vi "digital_demod_host.vi"() -> ()   [LabVIEW 2014]
uses:
  <vilib>/userdefined/High Color/nirio_resource_hc.ctl
  <vilib>/LabVIEW Targets/FPGA/RIO/nirio_PxiTriggers.ctl
  <vilib>/addons/h5labview2/file/H5Fmode.ctl
  <vilib>/FPGAPlugInAG/PXI-7854R/niLvFpga_Open_PXI-7854R.vi
  <vilib>/rvi/interface/common/dynamic/niFpgaDynamicAddResources.vi
  <vilib>/FPGAPlugInAG/Dynamic/niLvFpga_Run_Dynamic.vi
  <vilib>/LabVIEW Targets/FPGA/RIO/nirioReserveTrigger.vi
  <vilib>/Utility/error.llb/Error Cluster From Error Code.vi
  <vilib>/rvi/errors/niLvFpgaAdjustHostInterfaceError.vi
  <vilib>/addons/h5labview2/base/lib_path.vi
  <vilib>/addons/h5labview2/base/H5Equery.vi
  <vilib>/FPGAPlugInAG/Dynamic/niLvFpga_Close_Dynamic.vi
  <vilib>/rvi/interface/nirviOpenFPGA/nirviOpenFPGA.xnode
  FPGA Bitfiles/digitaldemod_FPGATarget_digitaldemodfpga_GJzl1kj7Fe4.lvbitx
  <vilib>/rvi/interface/nirviMethod/nirviMethod.xnode
  <vilib>/rvi/interface/nirviReadWriteControl/nirviReadWriteControl.xnode
  <vilib>/addons/h5labview2/base/hid_t.ctl
  <vilib>/addons/h5labview2/dataset/H5Dwrite.llb/H5Dwrite.xnode
  <vilib>/rvi/interface/nirviCloseFPGA/nirviCloseFPGA.xnode
  <vilib>/rvi/interface/Simulation/niFpgaSimulationCallBeginRW.vi
  <vilib>/rvi/errors/niLvFpgaMergeErrorWithErrorCode.vi
  <vilib>/FPGAPlugInAG/Dynamic/niLvFpga_ReadFifo_Dynamic.vi
  NiFpgaLv.dll
  <vilib>/addons/h5labview2/group/H5G.lvlib
  <vilib>/addons/h5labview2/file/H5F.lvlib
  <vilib>/FPGAPlugInAG/Dynamic/niLvFpga_StartFifo_Dynamic.vi
  <vilib>/FPGAPlugInAG/Dynamic/niLvFpga_StopFifo_Dynamic.vi
  National Instruments Downloads/LabVIEW FPGA English/FPGA Timekeeper 1.1b0/FPGA Timekeeper.lvlib
panel:
  in  "show_quad":bool
  out "delta_phi":cluster{dbl, dbl, dbl, dbl}(graph)
  in  "xy2_bitshift":i16
  in  "downsample->xyz":bool
  in  "inject_sigs":bool
  in  "Load last pars":bool
  in  "DAQ_trig":bool
  in  "Reset Phi 2":bool
  in  "reset_z_accum":bool
  out "config_trig":bool
  in  "block_hardware_trigs":bool=TRUE
  out "config_loaded":bool
  out "Nsamp_config":u32=50000
  out "fpga_dat_path":path=path "C:/Data/20180611/bead6/post_pump/turbombar_xyzcool_pumped_0_fpga.h5"
  in  "reset_trigs":bool
  in  "accept_trigs":bool
  out "amp4":dbl(graph)=1893.4088287353516
  out "phi4":dbl(graph)=0.028564453125
  in  "Change Pars 2":bool
  in  "xy_fb_bitshift":i16=-13
  in  "z_lower_lim":i16=-2000
  in  "z_upper_lim":i16=2000
  in  "z_fb_bitshift":i16=-16
  in  "z_ig":fxp<+/-,32,16>=-1.52587890625e-05
  in  "z_dg":fxp<+/-,32,16>=-0.0500640869140625
  in  "z_pg":fxp<+/-,32,16>=-0.0099945068359375
  in  "z_bitshift":i16
  in  "y_lower_lim":i16=-1000
  in  "y_upper_lim":i16=1000
  in  "y_dg":fxp<+/-,32,16>=-0.0019989013671875
  in  "x_lower_lim":i16=-1000
  in  "x_upper_lim":i16=1000
  in  "x_dg":fxp<+/-,32,16>=0.001007080078125
  in  "xy_bitshift":i16=-13
  in  "read_raw":bool
  out "z_fb":i16(graph)=-749
  out "z":i32(graph)=551
  out "y_fb":i16(graph)=2
  out "y":i32(graph)=-854
  out "x_fb":i16(graph)=-1
  out "x":i32(graph)=4640
  in  "z_set":fxp<+/-,32,32>
  in  "z_dc_offset":i16=-17500
  in  "y_dc_offset":i16
  in  "x_dc_offset":i16
  out "Host time (ns)":u64=1528843412913566976
  out "Target time (ns)":u64=1528843412913588017
  in  "downsamp_num":i16=100
  in  "Reset Phi Params":T1={"All Phi?"=TRUE, "Which?"=enum."0"}
  out "amp2":dbl(graph)=9755.388763427734
  out "amp3":dbl(graph)=9270.060470581055
  out "amp0":dbl(graph)=9360.88851928711
  out "amp1":dbl(graph)=10535.541046142578
  out "phi2":dbl(graph)=-7.1851806640625
  out "phi3":dbl(graph)=-7.253662109375
  in  "subtract_mean":bool=TRUE
  out "loop time":fxp<+,32,32>=2.0
  in  "Change Pars":bool
  out "phi0":dbl(graph)=-6.774658203125
  out "phi1":dbl(graph)=-6.8974609375
  in  "counter offset":u32
  in  "phase discont_neg":fxp<+/-,24,12>=-1.0
  in  "phase discont_pos":fxp<+/-,24,12>=1.0
  in  "Reset Phi":bool
  in  "loop timer (usec)":u32=2
  in  "Update ADC Clock":bool
  in  "Host Update Rate (msec)":dbl=1.0 format="%#_13g"
  in  "RIO Device":T2="RIO0"
  # "QPD AMPLITUDES"
  # "QPD PHASES"
  # "BACKSCATTER"
  # "BEAD XYZ + FB"
  # "X FEEDBACK"
  # "Y FEEDBACK"
  # "Z FEEDBACK"
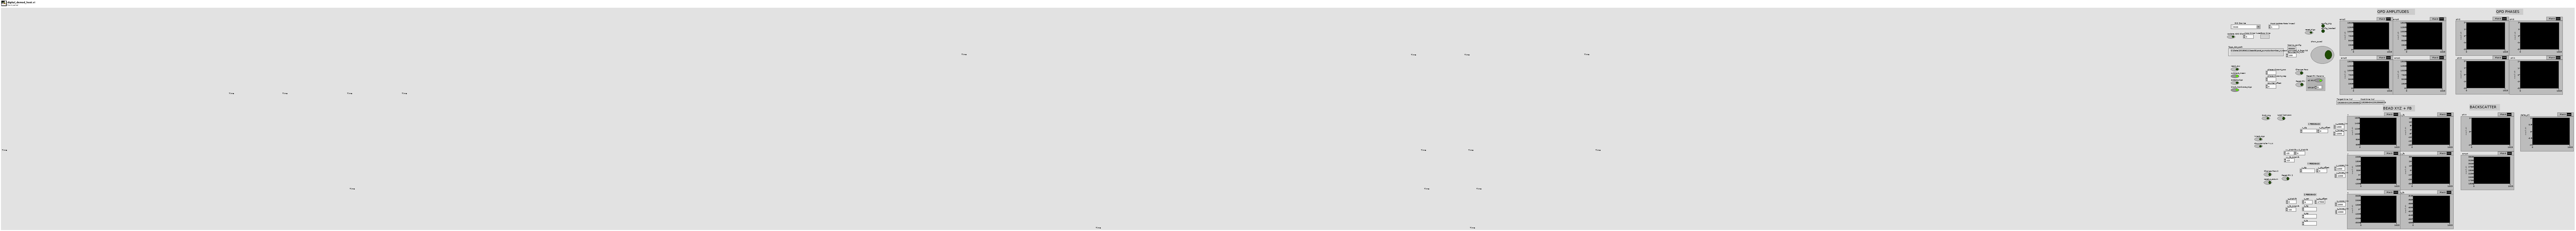
[diagram p1: front panel]
types:
  T1 = cluster{"All Phi?":bool, "Which?":enum16{"0", "1", "2", "3", "4"}}
  T2 = typedef "nirio_resource_hc.ctl" = tag
  T3 = typedef "nirio_PxiTriggers.ctl" = u16
  T4 = cluster{"phase discont_pos":fxp<+/-,24,12>, "phase discont_neg":fxp<+/-,24,12>, "counter offset":u32, "subtract_mean":bool, "downsamp_num":i16, "xy_bitshift":i16, "x_dg":fxp<+/-,32,16>, "x_upper_lim":i16, "x_lower_lim":i16, "x_dc_offset":i16, "y_dg":fxp<+/-,32,16>, "y_upper_lim":i16, "y_lower_lim":i16, "y_dc_offset":i16, "xy_fb_bitshift":i16, "z_bitshift":i16, "z_set":fxp<+/-,32,32>, "z_pg":fxp<+/-,32,16>, "z_dg":fxp<+/-,32,16>, "z_ig":fxp<+/-,32,16>, "z_fb_bitshift":i16, "z_upper_lim":i16, "z_lower_lim":i16, "z_dc_offset":i16, "inject_sigs":bool, "downsample->xyz":bool, "xy2_bitshift":i16}
  T5 = enum16{"open", "replace", "create", "open or create", "replace or create", "replace or create with confirmation"}
  T6 = typedef "H5F.lvlib/H5Fmode.ctl" = enum16{"read-only", "read-write", "overwrite", "create new", "open or create"}
  T7 = typedef "hid_t.ctl" = i32
  T8 = cluster{fxp<+/-,33,19>, fxp<+/-,33,19>, fxp<+/-,33,19>, fxp<+/-,33,19>}
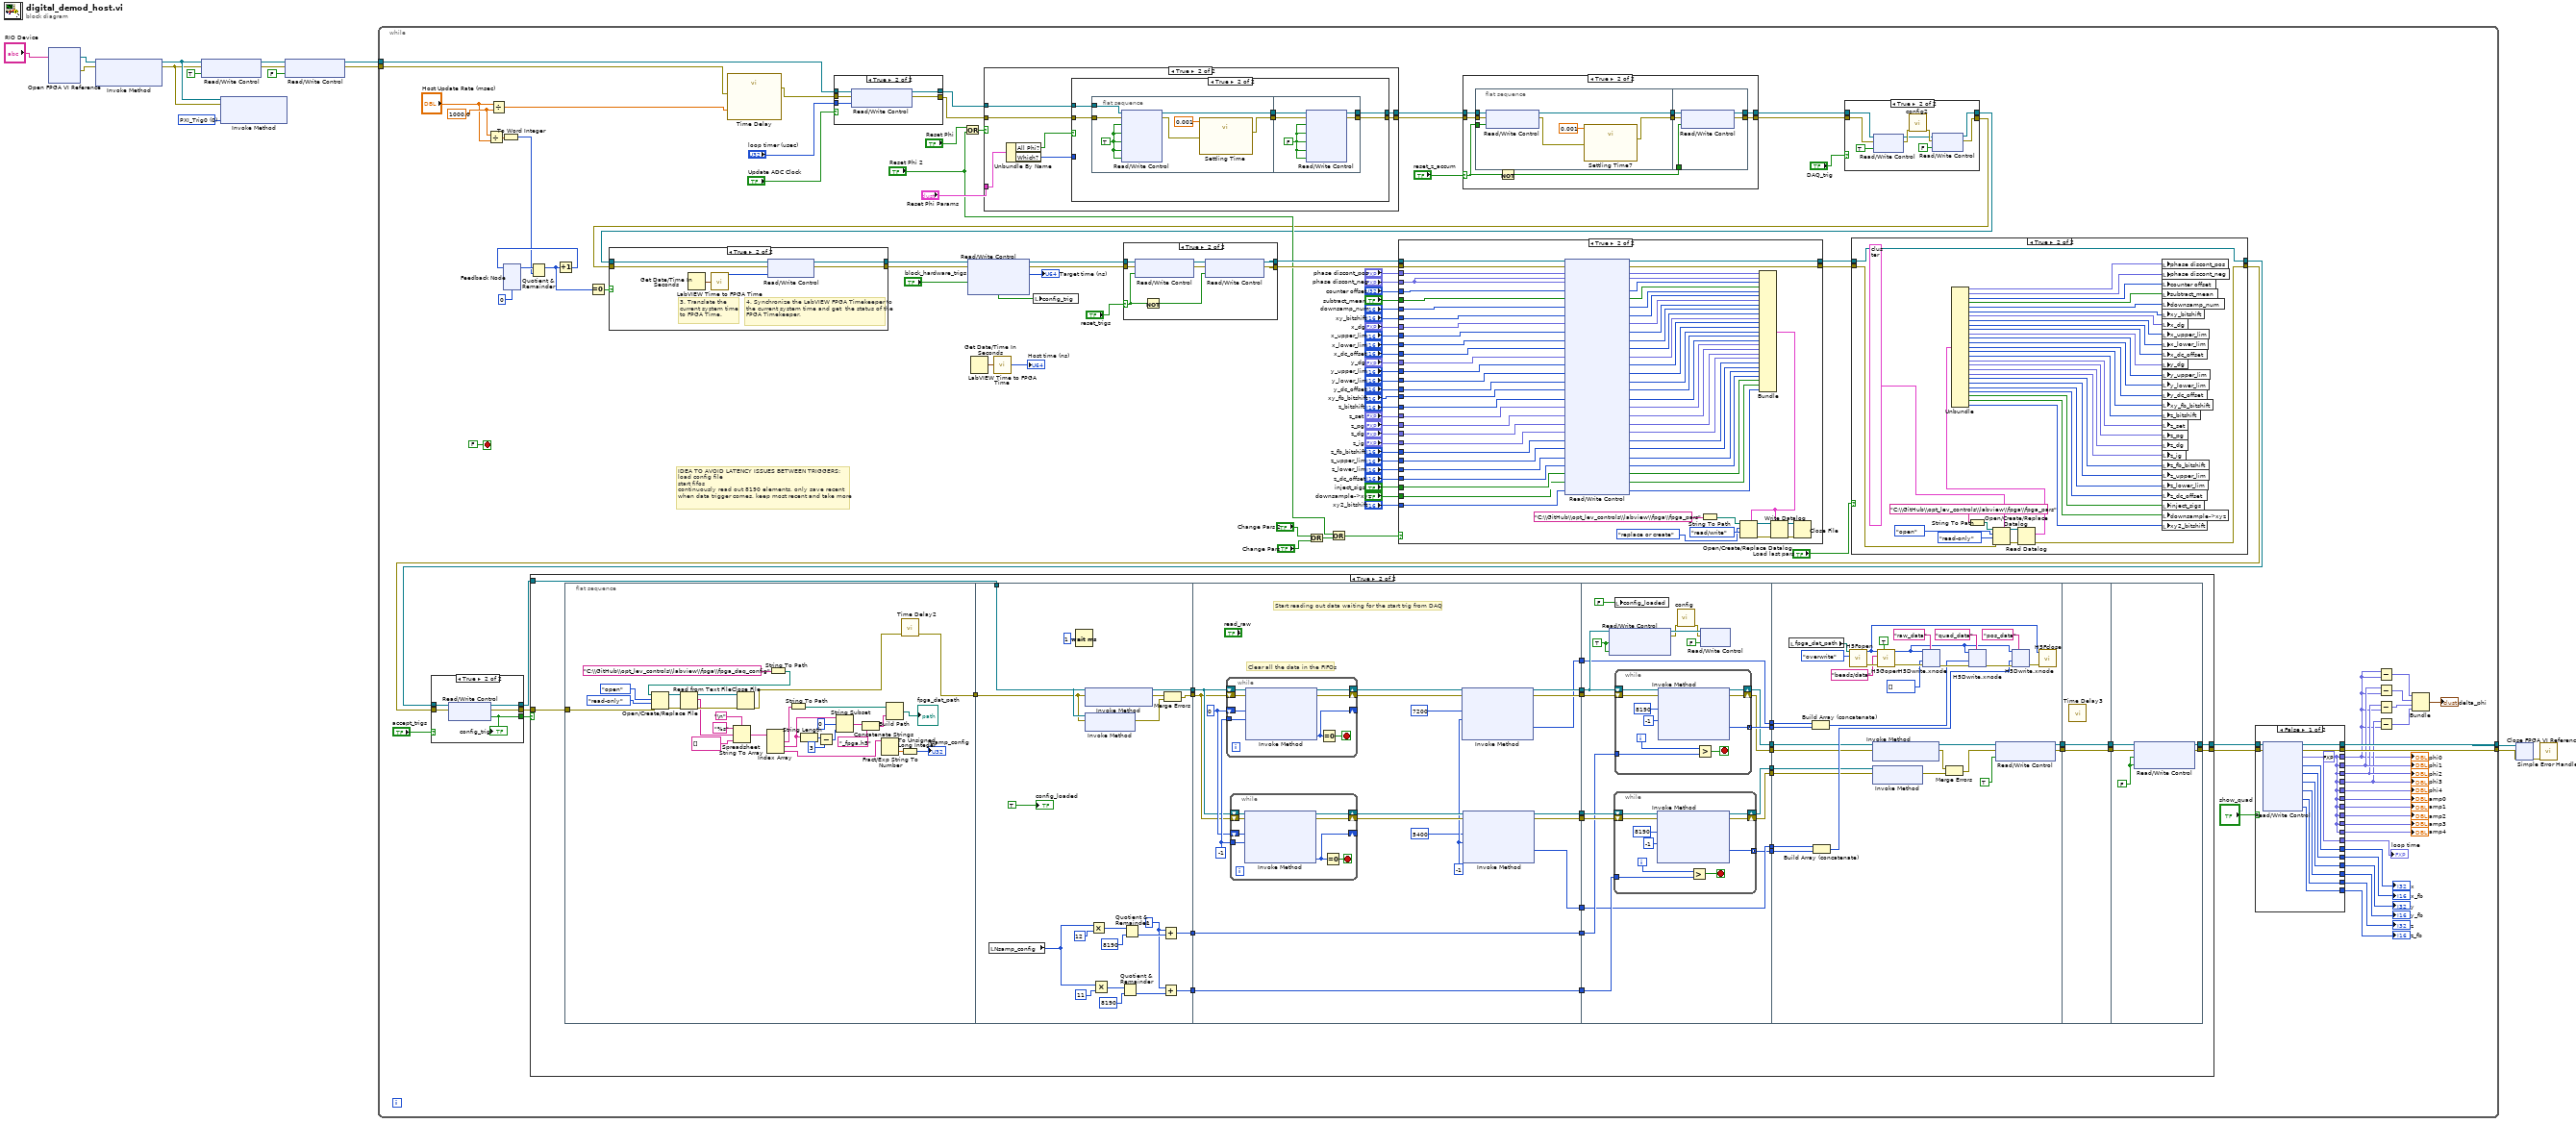
[diagram p0: block diagram]
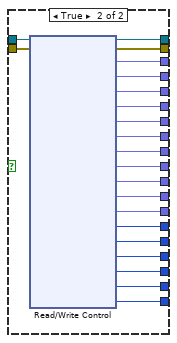
[diagram p2: hidden frame]
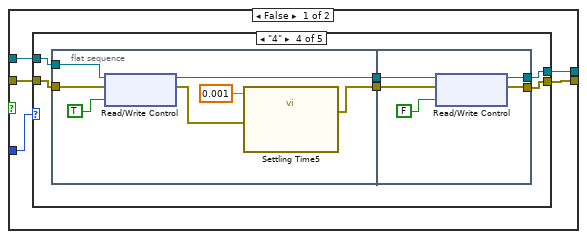
[diagram p12: hidden frame]
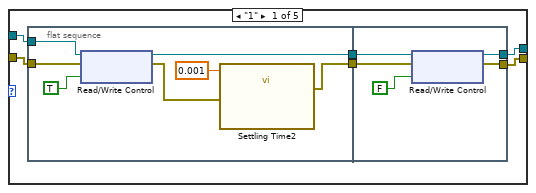
[diagram p13: hidden frame]
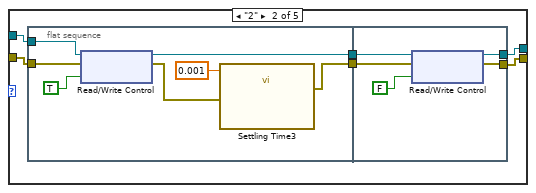
[diagram p14: hidden frame]
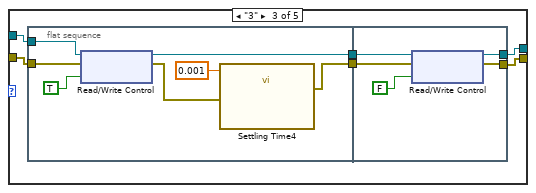
[diagram p15: hidden frame]
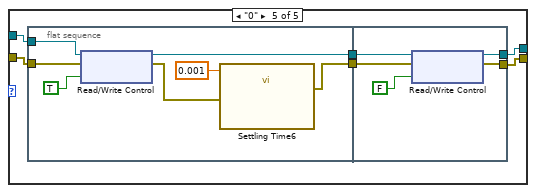
[diagram p16: hidden frame]
diagram:
  w1 = T3 0 items=["PXI_Trig0", "PXI_Trig1", "PXI_Trig2", "PXI_Trig3", "PXI_Trig4", "PXI_Trig5", "PXI_Trig6", "PXI_Trig7"] ("Trigger")
  n1 = xnode "Open FPGA VI Reference"("resource name"="RIO Device") -> ("FPGA VI Reference Out"=w11:refnum<k20>, "error out"=w10:errorcluster)  [unwired: 1 in]
  n2 = xnode "Invoke Method"("FPGA VI Reference In"=w11, "error in"=w10) -> ("FPGA VI Reference Out"=w3:refnum<k20>, "error out"=w2:errorcluster)  [unwired: 1 in]
  n3 = xnode "Read/Write Control"("FPGA VI Reference In"=w3, "error in"=w2, "reset_config_trig"=TRUE ("reset_trig")) -> ("FPGA VI Reference Out"=w6:refnum<k20>, "error out"=w4:errorcluster)
  n4 = xnode "Invoke Method"("FPGA VI Reference In"=w3, "error in"=w2, "Trigger"=w1) -> ()  [unwired: 2 out]
  n5 = xnode "Read/Write Control"("FPGA VI Reference In"=w6, "error in"=w4, "reset_config_trig"=FALSE ("manual_trig")) -> ("FPGA VI Reference Out"=w9:refnum<k20>, "error out"=w8:errorcluster)
  n6 = while {
    tunnel: w8 -> [w123]
    tunnel: w9 -> [w39]
    tunnel: [w114] -> w14
    tunnel: [w113] -> w13
    stop <- FALSE stop-if-true
    w104 = 1000.0
    # "IDEA TO AVOID LATENCY ISSUES BETWEEN TRIGGERS:\nload config file\nstart fifos\ncontinuously read out 8190 elements, only save recent\nwhen data trigger comes, keep most recent and take more"
    n7 = Divide(x=w104, y="Host Update Rate (msec)") -> (x/y=w102:dbl)
    n8 = Divide(x="Host Update Rate (msec)", y=w104) -> (x/y=w124:dbl)
    n9 = To Word Integer(number=w102) -> (16bit integer=w96:i16)
    n10 = feedback #1(i16 0) -> (w98:i16)
    n11 = Quotient & Remainder(x=w98, y=w96) -> (x-y*floor(x/y)=w95:i16)  [unwired: 1 out]
    n12 = Increment(x=w95) -> (x+1=w97:i16)
    n13 = feedback-in #1(w97) -> ()
    n14 = Equal To 0?(x=w95) -> (x = 0?=w100:bool)
    n15 = call "Time Delay"("error in (no error)"=w123, "Delay Time (s)"=w124) -> ("error out"=w121:errorcluster)  [unwired: 9 in]
    n16 = case shown="True" "Update ADC Clock" {
      tunnel: w39 -> [w671 w676]
      tunnel: w121 -> [w670 w675]
      tunnel: [w671 w674] -> w119
      tunnel: [w670 w673] -> w118
      tunnel: "loop timer (usec)" -> [_ w672]
      frame False {
      }
      frame True {
        n17 = xnode "Read/Write Control"("FPGA VI Reference In"=w676, "error in"=w675, "loop timer (usec)"=w672) -> ("FPGA VI Reference Out"=w674:refnum<k20>, "error out"=w673:errorcluster)
      }
    }
    n18 = Or(x="Reset Phi", y="Reset Phi 2") -> (x .or. y?=w45:bool)
    n19 = Get Date/Time In Seconds() -> (seconds since 1Jan1904=w93:timestamp)
    n20 = case shown="True" w45 {
      tunnel: w119 -> [w549 w556]
      tunnel: w118 -> [w548 w555]
      tunnel: [w549 w553] -> w48
      tunnel: [w548 w554] -> w47
      tunnel: "Reset Phi Params" -> [_ w552]
      frame False {
      }
      frame True {
        n21 = Unbundle By Name(w552) -> ("All Phi?"=w551:bool, "Which?"=w550:enum16{"0", "1", "2", "3", "4"})
        n22 = case shown="True" w551 {
          tunnel: w556 -> [w561 w655]
          tunnel: w555 -> [w560 w654]
          tunnel: [w558 w653] -> w554
          tunnel: [w559 w652] -> w553
          tunnel: w550 -> [w557 _]
          frame False {
            n23 = case shown="\"4\"" w557 {
              tunnel: w561 -> [w565 w583 w601 w619 w637]
              tunnel: w560 -> [w564 w582 w600 w618 w636]
              tunnel: [w563 w581 w599 w617 w635] -> w559
              tunnel: [w562 w580 w598 w616 w634] -> w558
              frame "1" {
                n24 = flat-sequence {
                  tunnel: w565 -> [w574]
                  tunnel: w564 -> [w573]
                  tunnel: [w572] -> w567
                  tunnel: [w569] -> w566
                  tunnel: w567 -> [w579]
                  tunnel: w566 -> [w578]
                  tunnel: [w577] -> w563
                  tunnel: [w576] -> w562
                  frame #0 {
                    n25 = xnode "Read/Write Control"("FPGA VI Reference In"=w574, "error in"=w573, "reset_phi1"=TRUE) -> ("FPGA VI Reference Out"=w572:refnum<k20>, "error out"=w570:errorcluster)
                    n26 = call "Settling Time2"("error in (no error)"=w570, "Delay Time (s)"=0.001) -> ("error out"=w569:errorcluster)  [unwired: 9 in]
                  }
                  frame #1 {
                    n27 = xnode "Read/Write Control"("FPGA VI Reference In"=w579, "error in"=w578, "reset_phi1"=FALSE) -> ("FPGA VI Reference Out"=w577:refnum<k20>, "error out"=w576:errorcluster)
                  }
                }
              }
              frame "2" {
                n28 = flat-sequence {
                  tunnel: w583 -> [w592]
                  tunnel: w582 -> [w591]
                  tunnel: [w590] -> w585
                  tunnel: [w587] -> w584
                  tunnel: w585 -> [w597]
                  tunnel: w584 -> [w596]
                  tunnel: [w595] -> w581
                  tunnel: [w594] -> w580
                  frame #0 {
                    n29 = xnode "Read/Write Control"("FPGA VI Reference In"=w592, "error in"=w591, "reset_phi2"=TRUE) -> ("FPGA VI Reference Out"=w590:refnum<k20>, "error out"=w588:errorcluster)
                    n30 = call "Settling Time3"("error in (no error)"=w588, "Delay Time (s)"=0.001) -> ("error out"=w587:errorcluster)  [unwired: 9 in]
                  }
                  frame #1 {
                    n31 = xnode "Read/Write Control"("FPGA VI Reference In"=w597, "error in"=w596, "reset_phi2"=FALSE) -> ("FPGA VI Reference Out"=w595:refnum<k20>, "error out"=w594:errorcluster)
                  }
                }
              }
              frame "3" {
                n32 = flat-sequence {
                  tunnel: w601 -> [w610]
                  tunnel: w600 -> [w609]
                  tunnel: [w608] -> w603
                  tunnel: [w605] -> w602
                  tunnel: w603 -> [w615]
                  tunnel: w602 -> [w614]
                  tunnel: [w613] -> w599
                  tunnel: [w612] -> w598
                  frame #0 {
                    n33 = xnode "Read/Write Control"("FPGA VI Reference In"=w610, "error in"=w609, "reset_phi3"=TRUE) -> ("FPGA VI Reference Out"=w608:refnum<k20>, "error out"=w606:errorcluster)
                    n34 = call "Settling Time4"("error in (no error)"=w606, "Delay Time (s)"=0.001) -> ("error out"=w605:errorcluster)  [unwired: 9 in]
                  }
                  frame #1 {
                    n35 = xnode "Read/Write Control"("FPGA VI Reference In"=w615, "error in"=w614, "reset_phi3"=FALSE) -> ("FPGA VI Reference Out"=w613:refnum<k20>, "error out"=w612:errorcluster)
                  }
                }
              }
              frame "4" {
                n36 = flat-sequence {
                  tunnel: w619 -> [w628]
                  tunnel: w618 -> [w627]
                  tunnel: [w626] -> w621
                  tunnel: [w623] -> w620
                  tunnel: w621 -> [w633]
                  tunnel: w620 -> [w632]
                  tunnel: [w631] -> w617
                  tunnel: [w630] -> w616
                  frame #0 {
                    n37 = xnode "Read/Write Control"("FPGA VI Reference In"=w628, "error in"=w627, "reset_phi4"=TRUE) -> ("FPGA VI Reference Out"=w626:refnum<k20>, "error out"=w624:errorcluster)
                    n38 = call "Settling Time5"("error in (no error)"=w624, "Delay Time (s)"=0.001) -> ("error out"=w623:errorcluster)  [unwired: 9 in]
                  }
                  frame #1 {
                    n39 = xnode "Read/Write Control"("FPGA VI Reference In"=w633, "error in"=w632, "reset_phi4"=FALSE) -> ("FPGA VI Reference Out"=w631:refnum<k20>, "error out"=w630:errorcluster)
                  }
                }
              }
              frame "0" {
                n40 = flat-sequence {
                  tunnel: w637 -> [w646]
                  tunnel: w636 -> [w645]
                  tunnel: [w644] -> w639
                  tunnel: [w641] -> w638
                  tunnel: w639 -> [w651]
                  tunnel: w638 -> [w650]
                  tunnel: [w649] -> w635
                  tunnel: [w648] -> w634
                  frame #0 {
                    n41 = xnode "Read/Write Control"("FPGA VI Reference In"=w646, "error in"=w645, "reset_phi0"=TRUE) -> ("FPGA VI Reference Out"=w644:refnum<k20>, "error out"=w642:errorcluster)
                    n42 = call "Settling Time6"("error in (no error)"=w642, "Delay Time (s)"=0.001) -> ("error out"=w641:errorcluster)  [unwired: 9 in]
                  }
                  frame #1 {
                    n43 = xnode "Read/Write Control"("FPGA VI Reference In"=w651, "error in"=w650, "reset_phi0"=FALSE) -> ("FPGA VI Reference Out"=w649:refnum<k20>, "error out"=w648:errorcluster)
                  }
                }
              }
            }
          }
          frame True {
            n44 = flat-sequence {
              tunnel: w655 -> [w664]
              tunnel: w654 -> [w663]
              tunnel: [w662] -> w657
              tunnel: [w659] -> w656
              tunnel: w657 -> [w669]
              tunnel: w656 -> [w668]
              tunnel: [w667] -> w652
              tunnel: [w666] -> w653
              frame #0 {
                w658 = TRUE
                n45 = xnode "Read/Write Control"("FPGA VI Reference In"=w664, "error in"=w663, "reset_phi0"=w658, "reset_phi1"=w658, "reset_phi2"=w658, "reset_phi3"=w658, "reset_phi4"=w658) -> ("FPGA VI Reference Out"=w662:refnum<k20>, "error out"=w660:errorcluster)
                n46 = call "Settling Time"("error in (no error)"=w660, "Delay Time (s)"=0.001) -> ("error out"=w659:errorcluster)  [unwired: 9 in]
              }
              frame #1 {
                w665 = FALSE
                n47 = xnode "Read/Write Control"("FPGA VI Reference In"=w669, "error in"=w668, "reset_phi0"=w665, "reset_phi1"=w665, "reset_phi2"=w665, "reset_phi3"=w665, "reset_phi4"=w665) -> ("FPGA VI Reference Out"=w667:refnum<k20>, "error out"=w666:errorcluster)
              }
            }
          }
        }
      }
    }
    n48 = call "LabVIEW Time to FPGA Time.vi"("LabVIEW time"=w93) -> ("FPGA time (ns)"=→"Host time (ns)":u64)
    n49 = Or(x="Change Pars 2", y="Change Pars") -> (x .or. y?=w43:bool)
    n50 = Or(x="Reset Phi 2", y=w43) -> (x .or. y?=w42:bool)
    n51 = case shown="True" "reset_z_accum" {
      selector: "reset_z_accum" -> [_ w212]
      tunnel: w48 -> [w210 w218]
      tunnel: w47 -> [w209 w217]
      tunnel: [w210 w216] -> w37
      tunnel: [w209 w215] -> w36
      frame False {
      }
      frame True {
        n52 = flat-sequence {
          tunnel: w218 -> [w225]
          tunnel: w217 -> [w224]
          tunnel: w212 -> [w222]
          tunnel: [w223] -> w214
          tunnel: [w219] -> w213
          tunnel: [w227] -> w215
          tunnel: [w228] -> w216
          tunnel: w214 -> [w230]
          tunnel: w213 -> [w229]
          tunnel: w211 -> [w226]
          frame #0 {
            n53 = xnode "Read/Write Control"("FPGA VI Reference In"=w225, "error in"=w224, "reset_z_accum"=w222) -> ("FPGA VI Reference Out"=w223:refnum<k20>, "error out"=w220:errorcluster)
            n54 = call "Settling Time7"("error in (no error)"=w220, "Delay Time (s)"=0.001) -> ("error out"=w219:errorcluster)  [unwired: 9 in]
          }
          frame #1 {
            n55 = xnode "Read/Write Control"("FPGA VI Reference In"=w230, "error in"=w229, "reset_z_accum"=w226) -> ("FPGA VI Reference Out"=w228:refnum<k20>, "error out"=w227:errorcluster)
          }
        }
        n56 = Not(x=w212) -> (.not. x?=w211:bool)
      }
    }
    n57 = case shown="True" "DAQ_trig" {
      tunnel: w37 -> [w199 w203]
      tunnel: w36 -> [w198 w202]
      tunnel: [w199 w201] -> w35
      tunnel: [w198 w200] -> w34
      frame False {
      }
      frame True {
        n58 = xnode "Read/Write Control"("FPGA VI Reference In"=w203, "error in"=w202, "TRIG0"=TRUE) -> ("FPGA VI Reference Out"=w205:refnum<k20>, "error out"=w206:errorcluster)
        n59 = call "config2"("error in (no error)"=w206) -> ("error out"=w207:errorcluster)  [unwired: 10 in]
        n60 = xnode "Read/Write Control"("FPGA VI Reference In"=w205, "error in"=w207, "TRIG0"=FALSE) -> ("FPGA VI Reference Out"=w201:refnum<k20>, "error out"=w200:errorcluster)
      }
    }
    n61 = case shown="True" w100 {
      tunnel: w34 -> [w498 w503]
      tunnel: w35 -> [w499 w502]
      tunnel: [w499 w501] -> w91
      tunnel: [w498 w500] -> w90
      frame False {
      }
      frame True {
        # "4. Synchronize the LabVIEW FPGA Timekeeper to the current system time and get  the status of the FPGA Timekeeper."
        # "3. Translate the current system time to FPGA Time."
        n62 = Get Date/Time In Seconds() -> (seconds since 1Jan1904=w505:timestamp)
        n63 = call "LabVIEW Time to FPGA Time.vi"("LabVIEW time"=w505) -> ("FPGA time (ns)"=w504:u64)
        n64 = xnode "Read/Write Control"("FPGA VI Reference In"=w502, "error in"=w503, "RT time (ns)"=w504) -> ("FPGA VI Reference Out"=w501:refnum<k20>, "error out"=w500:errorcluster)
      }
    }
    n65 = xnode "Read/Write Control"("FPGA VI Reference In"=w91, "error in"=w90, "block_config_trig"="block_hardware_trigs") -> ("FPGA VI Reference Out"=w60:refnum<k20>, "error out"=w59:errorcluster, "time (ns)"=→"Target time (ns)":u64, "config_trig"=w40:bool)
    n66 = local write "config_trig"(w40) -> ()
    n67 = case shown="True" "reset_trigs" {
      selector: "reset_trigs" -> [_ w491]
      tunnel: w60 -> [w489 w497]
      tunnel: w59 -> [w488 w496]
      tunnel: [w489 w493] -> w56
      tunnel: [w488 w492] -> w55
      frame False {
      }
      frame True {
        n68 = xnode "Read/Write Control"("FPGA VI Reference In"=w497, "error in"=w496, "reset_config_trig"=w491) -> ("FPGA VI Reference Out"=w495:refnum<k20>, "error out"=w494:errorcluster)
        n69 = Not(x=w491) -> (.not. x?=w490:bool)
        n70 = xnode "Read/Write Control"("FPGA VI Reference In"=w495, "error in"=w494, "reset_config_trig"=w490) -> ("FPGA VI Reference Out"=w493:refnum<k20>, "error out"=w492:errorcluster)
      }
    }
    n71 = case shown="True" w42 {
      tunnel: w55 -> [w507 w544]
      tunnel: [w507 w547] -> w31
      tunnel: [w506 w546] -> w33
      tunnel: w56 -> [w506 w545]
      tunnel: "phase discont_pos" -> [_ w543]
      tunnel: "phase discont_neg" -> [_ w542]
      tunnel: "counter offset" -> [_ w541]
      tunnel: "subtract_mean" -> [_ w540]
      tunnel: "downsamp_num" -> [_ w539]
      tunnel: "x_dc_offset" -> [_ w534]
      tunnel: "y_dc_offset" -> [_ w530]
      tunnel: "z_dc_offset" -> [_ w520]
      tunnel: "z_set" -> [_ w527]
      tunnel: "xy_bitshift" -> [_ w538]
      tunnel: "x_dg" -> [_ w537]
      tunnel: "x_upper_lim" -> [_ w536]
      tunnel: "x_lower_lim" -> [_ w535]
      tunnel: "y_dg" -> [_ w533]
      tunnel: "y_upper_lim" -> [_ w532]
      tunnel: "y_lower_lim" -> [_ w531]
      tunnel: "z_bitshift" -> [_ w528]
      tunnel: "z_pg" -> [_ w526]
      tunnel: "z_dg" -> [_ w525]
      tunnel: "z_ig" -> [_ w524]
      tunnel: "z_fb_bitshift" -> [_ w523]
      tunnel: "z_upper_lim" -> [_ w522]
      tunnel: "z_lower_lim" -> [_ w521]
      tunnel: "xy_fb_bitshift" -> [_ w529]
      tunnel: "inject_sigs" -> [_ w510]
      tunnel: "downsample->xyz" -> [_ w509]
      tunnel: "xy2_bitshift" -> [_ w508]
      frame False {
      }
      frame True {
        n72 = xnode "Read/Write Control"("FPGA VI Reference In"=w545, "error in"=w544, "discont_pos"=w543, "discont_neg"=w542, "Counter Offset"=w541, "subtract_mean"=w540, "downsamp_num"=w539, "xy_bitshift"=w538, "x_dg"=w537, "x_upper_lim"=w536, "x_lower_lim"=w535, "x_dc_offset"=w534, "y_dg"=w533, "y_upper_lim"=w532, "y_lower_lim"=w531, "y_dc_offset"=w530, "xy_fb_bitshift"=w529, "z_bitshift"=w528, "z_set"=w527, "z_pg"=w526, "z_dg"=w525, "z_ig"=w524, "z_fb_bitshift"=w523, "z_upper_lim"=w522, "z_lower_lim"=w521, "z_dc_offset"=w520, "inject_sigs"=w510, "downsample->xyz"=w509, "xy2_bitshift"=w508) -> ("FPGA VI Reference Out"=w546:refnum<k20>, "error out"=w547:errorcluster)
        n73 = String To Path(string="C:\\GitHub\\opt_lev_controls\\labview\\fpga\\fpga_pars") -> (path=w512:path)
        n74 = Bundle("phase discont_pos"=w543, "phase discont_neg"=w542, "counter offset"=w541, "subtract_mean"=w540, "downsamp_num"=w539, "xy_bitshift"=w538, "x_dg"=w537, "x_upper_lim"=w536, "x_lower_lim"=w535, "x_dc_offset"=w534, "y_dg"=w533, "y_upper_lim"=w532, "y_lower_lim"=w531, "y_dc_offset"=w530, "xy_fb_bitshift"=w529, "z_bitshift"=w528, "z_set"=w527, "z_pg"=w526, "z_dg"=w525, "z_ig"=w524, "z_fb_bitshift"=w523, "z_upper_lim"=w522, "z_lower_lim"=w521, "z_dc_offset"=w520, "inject_sigs"=w510, "downsample->xyz"=w509, "xy2_bitshift"=w508) -> (w515:T4)  [unwired: 1 in]
        n75 = Open/Create/Replace Datalog(5:w515, 9:enum16{"read/write", "read-only", "write-only"}."read/write" ("access (0:read/write)"), 10:T5."replace or create" ("operation (0:open)"), 11:w512) -> (0:w519:errorcluster, 3:w517:refnum<k1>)  [unwired: 2 in, 1 out]
        n76 = Write Datalog(4:w519, 6:w515, 7:w517) -> (0:w518:errorcluster, 3:w516:refnum<k1>)
        n77 = Close File(refnum=w516, error in=w518) -> ()  [unwired: 2 out]
      }
    }
    n78 = case shown="True" "Load last pars" {
      tunnel: [w159 w193] -> w32
      tunnel: w33 -> [w159 w193]
      tunnel: [w158 w180] -> w30
      tunnel: w31 -> [w158 w194]
      frame False {
      }
      frame True {
        n79 = String To Path(string="C:\\GitHub\\opt_lev_controls\\labview\\fpga\\fpga_pars") -> (path=w197:path)
        n80 = Open/Create/Replace Datalog(5:T4 {"phase discont_pos"=0.0, "phase discont_neg"=0.0, "counter offset"=0, "subtract_mean"=FALSE, "downsamp_num"=0, "xy_bitshift"=0, "x_dg"=0.0, "x_upper_lim"=0, "x_lower_lim"=0, "x_dc_offset"=0, "y_dg"=0.0, "y_upper_lim"=0, "y_lower_lim"=0, "y_dc_offset"=0, "xy_fb_bitshift"=0, "z_bitshift"=0, "z_set"=0.0, "z_pg"=0.0, "z_dg"=0.0, "z_ig"=0.0, "z_fb_bitshift"=0, "z_upper_lim"=0, "z_lower_lim"=0, "z_dc_offset"=0, "inject_sigs"=FALSE, "downsample->xyz"=FALSE, "xy2_bitshift"=0} ("output cluster"), 8:w194, 9:enum16{"read/write", "read-only", "write-only"}."read-only" ("access (0:read/write)"), 10:T5."open" ("operation (0:open)"), 11:w197) -> (0:w191:errorcluster, 3:w192:refnum<k1>)  [unwired: 1 in, 1 out]
        n81 = Read Datalog(4:w191, 7:w192) -> (0:w180:errorcluster, 2:w190:T4)  [unwired: 1 in, 1 out]
        n82 = Unbundle(w190) -> ("phase discont_pos"=w189:fxp<+/-,24,12>, "phase discont_neg"=w188:fxp<+/-,24,12>, "counter offset"=w187:u32, "subtract_mean"=w186:bool, "downsamp_num"=w185:i16, "xy_bitshift"=w184:i16, "x_dg"=w183:fxp<+/-,32,16>, "x_upper_lim"=w182:i16, "x_lower_lim"=w181:i16, "x_dc_offset"=w179:i16, "y_dg"=w178:fxp<+/-,32,16>, "y_upper_lim"=w177:i16, "y_lower_lim"=w176:i16, "y_dc_offset"=w175:i16, "xy_fb_bitshift"=w174:i16, "z_bitshift"=w173:i16, "z_set"=w172:fxp<+/-,32,32>, "z_pg"=w171:fxp<+/-,32,16>, "z_dg"=w170:fxp<+/-,32,16>, "z_ig"=w169:fxp<+/-,32,16>, "z_fb_bitshift"=w168:i16, "z_upper_lim"=w167:i16, "z_lower_lim"=w166:i16, "z_dc_offset"=w165:i16, "inject_sigs"=w162:bool, "downsample->xyz"=w161:bool, "xy2_bitshift"=w160:i16)
        n83 = local write "phase discont_pos"(w189) -> ()
        n84 = local write "phase discont_neg"(w188) -> ()
        n85 = local write "counter offset"(w187) -> ()
        n86 = local write "subtract_mean"(w186) -> ()
        n87 = local write "downsamp_num"(w185) -> ()
        n88 = local write "xy_bitshift"(w184) -> ()
        n89 = local write "x_dg"(w183) -> ()
        n90 = local write "x_upper_lim"(w182) -> ()
        n91 = local write "x_lower_lim"(w181) -> ()
        n92 = local write "x_dc_offset"(w179) -> ()
        n93 = local write "y_dg"(w178) -> ()
        n94 = local write "y_upper_lim"(w177) -> ()
        n95 = local write "y_lower_lim"(w176) -> ()
        n96 = local write "y_dc_offset"(w175) -> ()
        n97 = local write "xy_fb_bitshift"(w174) -> ()
        n98 = local write "z_bitshift"(w173) -> ()
        n99 = local write "z_set"(w172) -> ()
        n100 = local write "z_pg"(w171) -> ()
        n101 = local write "z_dg"(w170) -> ()
        n102 = local write "z_ig"(w169) -> ()
        n103 = local write "z_fb_bitshift"(w168) -> ()
        n104 = local write "z_upper_lim"(w167) -> ()
        n105 = local write "z_lower_lim"(w166) -> ()
        n106 = local write "z_dc_offset"(w165) -> ()
        n107 = local write "inject_sigs"(w162) -> ()
        n108 = local write "downsample->xyz"(w161) -> ()
        n109 = local write "xy2_bitshift"(w160) -> ()
      }
    }
    n110 = case shown="True" "accept_trigs" {
      selector: "accept_trigs" -> [w233 _]
      tunnel: [w233 w238] -> w54
      tunnel: w30 -> [w231 w237]
      tunnel: w32 -> [w232 w236]
      tunnel: [w232 w235] -> w51
      tunnel: [w231 w234] -> w50
      frame False {
      }
      frame True {
        n111 = xnode "Read/Write Control"("FPGA VI Reference In"=w236, "error in"=w237) -> ("FPGA VI Reference Out"=w235:refnum<k20>, "error out"=w234:errorcluster, "config_trig"=w238:bool)
        "config_trig" <- w238
      }
    }
    n112 = case shown="True" w54 {
      tunnel: w51 -> [w240 w268]
      tunnel: [w240 w247] -> w53
      tunnel: [w239 w246] -> w52
      tunnel: w50 -> [w239 w245]
      frame False {
      }
      frame True {
        n113 = flat-sequence {
          tunnel: [w270] -> w269
          tunnel: w245 -> [w272]
          tunnel: w269 -> [w300]
          tunnel: w268 -> [w301]
          tunnel: [w306] -> w267
          tunnel: [w303] -> w266
          tunnel: [w305] -> w260
          tunnel: [w304] -> w258
          tunnel: w267 -> [w324]
          tunnel: w266 -> [w325]
          tunnel: [w335] -> w265
          tunnel: [w334] -> w264
          tunnel: [w328] -> w263
          tunnel: [w327] -> w262
          tunnel: [w333] -> w261
          tunnel: w260 -> [w333]
          tunnel: [w332] -> w259
          tunnel: w258 -> [w332]
          tunnel: [w331] -> w256
          tunnel: [w326] -> w253
          tunnel: w265 -> [w369]
          tunnel: w264 -> [w374]
          tunnel: w263 -> [w373]
          tunnel: w262 -> [w372]
          tunnel: w261 -> [w371]
          tunnel: w259 -> [w370]
          tunnel: [w368] -> w257
          tunnel: w256 -> [w368]
          tunnel: [w367] -> w255
          tunnel: [w366] -> w254
          tunnel: w253 -> [w366]
          tunnel: [w365] -> w252
          tunnel: [w364] -> w251
          tunnel: [w363] -> w250
          tunnel: [w362] -> w249
          tunnel: [w361] -> w248
          tunnel: w257 -> [w407]
          tunnel: w255 -> [w406]
          tunnel: w254 -> [w405]
          tunnel: w252 -> [w404]
          tunnel: w251 -> [w401]
          tunnel: w250 -> [w400]
          tunnel: w249 -> [w398]
          tunnel: w248 -> [w399]
          tunnel: [w397] -> w244
          tunnel: [w396] -> w242
          tunnel: w244 -> [w482]
          tunnel: [w482] -> w243
          tunnel: w242 -> [w481]
          tunnel: [w481] -> w241
          tunnel: [w484] -> w246
          tunnel: [w485] -> w247
          tunnel: w243 -> [w487]
          tunnel: w241 -> [w486]
          frame #0 {
            n114 = String To Path(string="C:\\GitHub\\opt_lev_controls\\labview\\fpga\\fpga_daq_config") -> (path=w298:path)
            n115 = Open/Create/Replace File(file path (use dialog)=w298, error in=w272, operation (0:open)=T5."open", access (0:read/write)=enum16{"read/write", "read-only", "write-only"}."read-only") -> (refnum out=w295:refnum<file>, error out=w294:errorcluster)  [unwired: 2 in, 1 out]
            n116 = Read from Text File(file (use dialog)=w295, error in=w294) -> (refnum out=w293:refnum<file>, text=w291:string, error out=w292:errorcluster)  [unwired: 2 in, 1 out]
            n117 = Spreadsheet String To Array(delimiter (Tab)="\n", format string="%s", spreadsheet string=w291, array type (2D Dbl)=string[] [] ("array of strings")) -> (array=w287:string[])
            n118 = Close File(refnum=w293, error in=w292) -> (error out=w271:errorcluster)  [unwired: 1 out]
            n119 = Index Array(array=w287) -> (element #1=w286:string, element #2=w283:string, element #3=w275:string)  [unwired: 3 in]
            n120 = String To Path(string=w286) -> (path=w285:path)
            n121 = String Length(string=w283) -> (length=w282:i32)
            n122 = Subtract(x=w282, y=3) -> (x-y=w280:i32)
            n123 = String Subset(string=w283, offset (0)=0, length (rest)=w280) -> (substring=w279:string)
            n124 = Concatenate Strings(w279, "_fpga.h5" ("string")) -> (w277:string)
            n125 = Fract/Exp String To Number(string=w275) -> (number=w274:dbl)  [unwired: 3 in, 1 out]
            n126 = Build Path(base path=w285, name or relative path=w277) -> (appended path=→"fpga_dat_path":path)
            n127 = To Unsigned Long Integer(number=w274) -> (unsigned 32bit integer=→"Nsamp_config":u32)
            n128 = call "Time Delay2"("error in (no error)"=w271) -> ("error out"=w270:errorcluster)  [unwired: 10 in]
          }
          frame #1 {
            w313 = u32 1 ("Extra Samps")
            n129 = local read "Nsamp_config"() -> (w311:u32)
            n130 = Wait (ms)(milliseconds to wait=u32 1) -> ()  [unwired: 1 out]
            n131 = xnode "Invoke Method"("FPGA VI Reference In"=w301, "error in"=w300) -> ("error out"=w308:errorcluster)  [unwired: 1 out]
            n132 = xnode "Invoke Method"("FPGA VI Reference In"=w301, "error in"=w300) -> ("FPGA VI Reference Out"=w303:refnum<k20>, "error out"=w307:errorcluster)
            n133 = Multiply(x=w311, y=u32 12) -> (x*y=w310:u32)
            n134 = Multiply(x=w311, y=u32 11) -> (x*y=w309:u32)
            n135 = Quotient & Remainder(x=w309, y=u32 8190) -> (floor(x/y)=w314:u32)  [unwired: 1 out]
            n136 = Quotient & Remainder(x=w310, y=u32 8190) -> (floor(x/y)=w316:u32)  [unwired: 1 out]
            n137 = Add(x=w313, y=w316) -> (x+y=w305:u32)
            n138 = Add(x=w313, y=w314) -> (x+y=w304:u32)
            n139 = Merge Errors(w307, w308) -> (w306:errorcluster)
            "config_loaded" <- TRUE
          }
          frame #2 {
            w323 = -1 ("Timeout (ms)")
            w337 = u32 0 ("Elements Remaining")
            w338 = -1
            # "Start reading out data waiting for the start trig from DAQ"
            # "Clear all the data in the FIFOs"
            n140 = while {
              tunnel: w338 -> [w349]
              shift-right: [w351] -> w336
              shift-left: w325 -> [w354]
              shift-right: [w350] -> w322
              shift-left: w324 -> [w353]
              shift-right: [w348] -> _
              shift-left: w337 -> [w352]
              stop <- w347 stop-if-true
              n141 = xnode "Invoke Method"("FPGA VI Reference In"=w354, "error in"=w353, "Number of Elements"=w352, "Timeout (ms)"=w349) -> ("FPGA VI Reference Out"=w351:refnum<k20>, "error out"=w350:errorcluster, "Elements Remaining"=w348:u32)  [unwired: 1 out]
              n142 = Equal To 0?(x=w348) -> (x = 0?=w347:bool)
            }
            n143 = while {
              tunnel: w338 -> [w341]
              shift-right: [w343] -> w330
              shift-left: w325 -> [w346]
              shift-right: [w342] -> w329
              shift-left: w324 -> [w345]
              shift-right: [w340] -> _
              shift-left: w337 -> [w344]
              stop <- w339 stop-if-true
              n144 = xnode "Invoke Method"("FPGA VI Reference In"=w346, "error in"=w345, "Number of Elements"=w344, "Timeout (ms)"=w341) -> ("FPGA VI Reference Out"=w343:refnum<k20>, "error out"=w342:errorcluster, "Elements Remaining"=w340:u32)  [unwired: 1 out]
              n145 = Equal To 0?(x=w340) -> (x = 0?=w339:bool)
            }
            n146 = xnode "Invoke Method"("FPGA VI Reference In"=w336, "error in"=w322, "Number of Elements"=u32 7200, "Timeout (ms)"=w323) -> ("FPGA VI Reference Out"=w335:refnum<k20>, "error out"=w334:errorcluster, "Data"=w331:i32[])  [unwired: 1 out]
            n147 = xnode "Invoke Method"("FPGA VI Reference In"=w330, "error in"=w329, "Number of Elements"=u32 5400, "Timeout (ms)"=w323) -> ("FPGA VI Reference Out"=w328:refnum<k20>, "error out"=w327:errorcluster, "Data"=w326:i32[])  [unwired: 1 out]
          }
          frame #3 {
            w359 = TRUE
            n148 = xnode "Read/Write Control"("FPGA VI Reference In"=w369, "block_config_trig"=w359, "TRIG0"=w359) -> ("FPGA VI Reference Out"=w358:refnum<k20>, "error out"=w357:errorcluster)  [unwired: 1 in]
            n149 = while {
              shift-right: [w380] -> w362
              shift-left: w373 -> [w384]
              shift-right: [w379] -> w361
              shift-left: w372 -> [w383]
              tunnel: w370 -> [w376]
              tunnel: [w375] -> w365 mode=concatenating
              i -> [w378]
              stop <- w377 stop-if-true
              n150 = xnode "Invoke Method"("FPGA VI Reference In"=w384, "error in"=w383, "Number of Elements"=u32 8190, "Timeout (ms)"=-1) -> ("FPGA VI Reference Out"=w380:refnum<k20>, "error out"=w379:errorcluster, "Data"=w375:i32[])  [unwired: 1 out]
              n151 = Greater?(x=w378, y=w376) -> (0:w377:bool)
            }
            n152 = local write "config_loaded"(FALSE) -> ()
            n153 = while {
              shift-right: [w390] -> w364
              shift-left: w369 -> [w394]
              shift-right: [w389] -> w363
              shift-left: w374 -> [w393]
              tunnel: w371 -> [w386]
              tunnel: [w385] -> w367 mode=concatenating
              i -> [w388]
              stop <- w387 stop-if-true
              n154 = xnode "Invoke Method"("FPGA VI Reference In"=w394, "error in"=w393, "Number of Elements"=u32 8190, "Timeout (ms)"=-1) -> ("FPGA VI Reference Out"=w390:refnum<k20>, "error out"=w389:errorcluster, "Data"=w385:i32[])  [unwired: 1 out]
              n155 = Greater?(x=w388, y=w386) -> (0:w387:bool)
            }
            n156 = call "config"("error in (no error)"=w357) -> ("error out"=w356:errorcluster)  [unwired: 10 in]
            n157 = xnode "Read/Write Control"("FPGA VI Reference In"=w358, "error in"=w356, "TRIG0"=FALSE) -> ()  [unwired: 2 out]
          }
          frame #4 {
            n158 = local read "fpga_dat_path"() -> (w412:path)
            n159 = Build Array (concatenate)(w407, w406) -> (w403:i32[])
            n160 = Build Array (concatenate)(w405, w404) -> (w402:i32[])
            n161 = call <vilib>:"H5Fopen.vi"("mode (read-only)"=H5Fmode."overwrite", "path"=w412) -> ("error out"=w416:errorcluster, "ref out"=w409:T7)  [unwired: 8 in]
            n162 = xnode "Invoke Method"("FPGA VI Reference In"=w401, "error in"=w400) -> ("FPGA VI Reference Out"=w418:refnum<k20>, "error out"=w423:errorcluster)
            n163 = xnode "Invoke Method"("FPGA VI Reference In"=w398, "error in"=w399) -> ("error out"=w422:errorcluster)  [unwired: 1 out]
            n164 = call <vilib>:"H5Gopen.vi"("create? (F)"=TRUE, "error in (no error)"=w416, "name"="beads/data", "ref in"=w409) -> ("error out"=w410:errorcluster, "group out"=w411:T7)  [unwired: 6 in]
            n165 = xnode "H5Dwrite.xnode"("dataset name"="raw_data", "error in (no error)"=w410, "data"=u64[] [], "ref in"=w411) -> ("error out"=w425:errorcluster)  [unwired: 3 in, 2 out]
            n166 = Merge Errors(w423, w422) -> (w395:errorcluster)
            n167 = xnode "H5Dwrite.xnode"("dataset name"="quad_data", "error in (no error)"=w425, "data"=w403, "ref in"=w411) -> ("error out"=w421:errorcluster)  [unwired: 3 in, 2 out]
            n168 = xnode "Read/Write Control"("FPGA VI Reference In"=w418, "error in"=w395, "reset_config_trig"=TRUE) -> ("FPGA VI Reference Out"=w397:refnum<k20>, "error out"=w396:errorcluster)
            n169 = xnode "H5Dwrite.xnode"("dataset name"="pos_data", "error in (no error)"=w421, "data"=w402, "ref in"=w411) -> ("error out"=w420:errorcluster)  [unwired: 3 in, 2 out]
            n170 = call <vilib>:"H5Fclose.vi"("error in (no error)"=w420, "ref"=w409) -> ()  [unwired: 9 in, 1 out]
          }
          frame #5 {
            n171 = call "Time Delay3"() -> ()  [unwired: 11 in, 1 out]
          }
          frame #6 {
            w483 = FALSE
            n172 = xnode "Read/Write Control"("FPGA VI Reference In"=w487, "error in"=w486, "block_config_trig"=w483, "reset_config_trig"=w483) -> ("FPGA VI Reference Out"=w485:refnum<k20>, "error out"=w484:errorcluster)
          }
        }
      }
    }
    n173 = case shown="False" "show_quad" {
      tunnel: [w134 w157] -> w114
      tunnel: [w133 w156] -> w113
      tunnel: [w132 w155] -> w111
      tunnel: [w125 w154] -> w110
      tunnel: [w125 w153] -> w109
      tunnel: [w125 w152] -> w108
      tunnel: [w125 w151] -> w107
      tunnel: [w131 w150] -> w85
      tunnel: [w130 w149] -> w84
      tunnel: [w129 w148] -> w83
      tunnel: [w128 w147] -> w82
      tunnel: [w127 w146] -> w81
      tunnel: [w126 w145] -> w80
      tunnel: [w125 w144] -> w62
      tunnel: [w125 w143] -> w61
      tunnel: w53 -> [w136 w142]
      tunnel: w52 -> [w135 w141]
      tunnel: [w125 w140] -> w25
      tunnel: [w125 w139] -> w24
      tunnel: [w125 w138] -> w23
      tunnel: [w125 w137] -> w22
      frame False {
        w125 = fxp<+/-,32,18> 0.0 ("phi0_full_out")
        n174 = xnode "Read/Write Control"("FPGA VI Reference In"=w136, "error in"=w135) -> ("FPGA VI Reference Out"=w134:refnum<k20>, "error out"=w133:errorcluster, "loop time"=w132:fxp<+,32,32>, "x_shifted"=w131:i32, "x_fb_i16"=w130:i16, "y_shifted"=w129:i32, "y_fb_i16"=w128:i16, "z_shifted"=w127:i32, "z_fb_i16"=w126:i16)
      }
      frame True {
        n175 = xnode "Read/Write Control"("FPGA VI Reference In"=w142, "error in"=w141) -> ("FPGA VI Reference Out"=w157:refnum<k20>, "error out"=w156:errorcluster, "phi0_full_out"=w137:fxp<+/-,32,18>, "phi1_full_out"=w140:fxp<+/-,32,18>, "phi2_full_out"=w139:fxp<+/-,32,18>, "phi3_full_out"=w138:fxp<+/-,32,18>, "phi4_full_out"=w144:fxp<+/-,32,18>, "amp0_out"=w151:fxp<+,32,16>, "amp1_out"=w152:fxp<+,32,16>, "amp2_out"=w153:fxp<+,32,16>, "amp3_out"=w154:fxp<+,32,16>, "amp4_out"=w143:fxp<+,32,16>, "loop time"=w155:fxp<+,32,32>, "x_shifted"=w150:i32, "x_fb_i16"=w149:i16, "y_shifted"=w148:i32, "y_fb_i16"=w147:i16, "z_shifted"=w146:i32, "z_fb_i16"=w145:i16)
      }
    }
    "phi1" <- w25
    "phi0" <- w22
    "loop time" <- w111
    "phi3" <- w23
    "phi2" <- w24
    "amp1" <- w108
    "amp0" <- w107
    "amp3" <- w110
    "amp2" <- w109
    "x" <- w85
    "x_fb" <- w84
    "y" <- w83
    "y_fb" <- w82
    "z" <- w81
    "z_fb" <- w80
    "phi4" <- w62
    "amp4" <- w61
    n176 = Subtract(x=w22, y=w22) -> (x-y=w21:fxp<+/-,33,19>)
    n177 = Subtract(x=w25, y=w22) -> (x-y=w20:fxp<+/-,33,19>)
    n178 = Subtract(x=w24, y=w22) -> (x-y=w19:fxp<+/-,33,19>)
    n179 = Subtract(x=w23, y=w22) -> (x-y=w18:fxp<+/-,33,19>)
    n180 = Bundle(w21, w20, w19, w18) -> (→"delta_phi":T8)  [unwired: 1 in]
  }
  n181 = xnode "Close FPGA VI Reference"("FPGA VI Reference In"=w14, "error in"=w13) -> ("error out"=w15:errorcluster)
  n182 = call <vilib>:"Simple Error Handler.vi"("error in (no error)"=w15) -> ()  [unwired: 4 in, 5 out]
